vi "Execute.vi"(8 "error in (no error)":errorcluster, 10 "ObserverRegistry in":refnum<class "ObserverRegistry.lvclass">, 11 "ObserverRegistryCommand":refnum<class "Observer_RegisterForErrors.lvclass">) -> (0 "error out":errorcluster, 2 "ObserverRegistry out":refnum<class "ObserverRegistry.lvclass">, 3 "Message":refnum<class "MSG.lvclass">)   [LabVIEW 2011, in "Messenging.lvlib" / "Observer_RegisterForErrors.lvclass"]
uses:
  Observer_RegisterForErrors.lvclass
  ObserverRegistry.lvclass
  Interprocess Messenger/TextVarientMessage/MSG.lvclass
  Interprocess Messenger/SendMultiple/Create Observer.vi
  ParentCommand/ObserverRegistryCommand.lvclass
  Messenging.lvlib
  Interprocess Messenger/SendMultiple/ObserverSet.lvclass
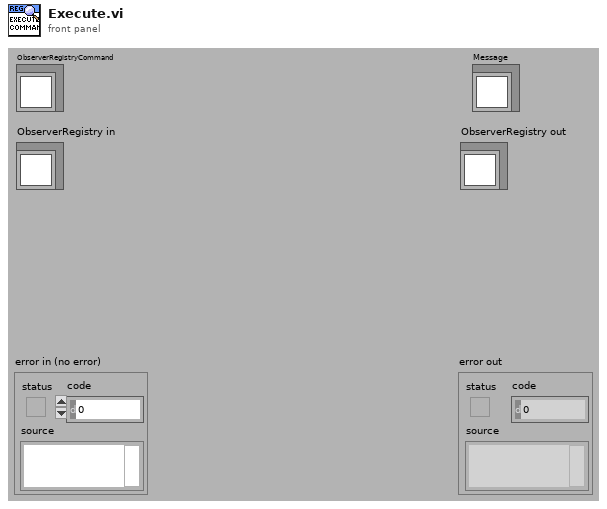
[diagram p1: front panel]
types:
  T1 = typedef "Messenging.lvlib/ObserverRegistry.lvclass/ObserverRegistryData.ctl" = cluster{"Observer of Errors":refnum<class "Observer.lvclass">, "Observer of All":refnum<class "Observer.lvclass">, "Event Registry":variant}
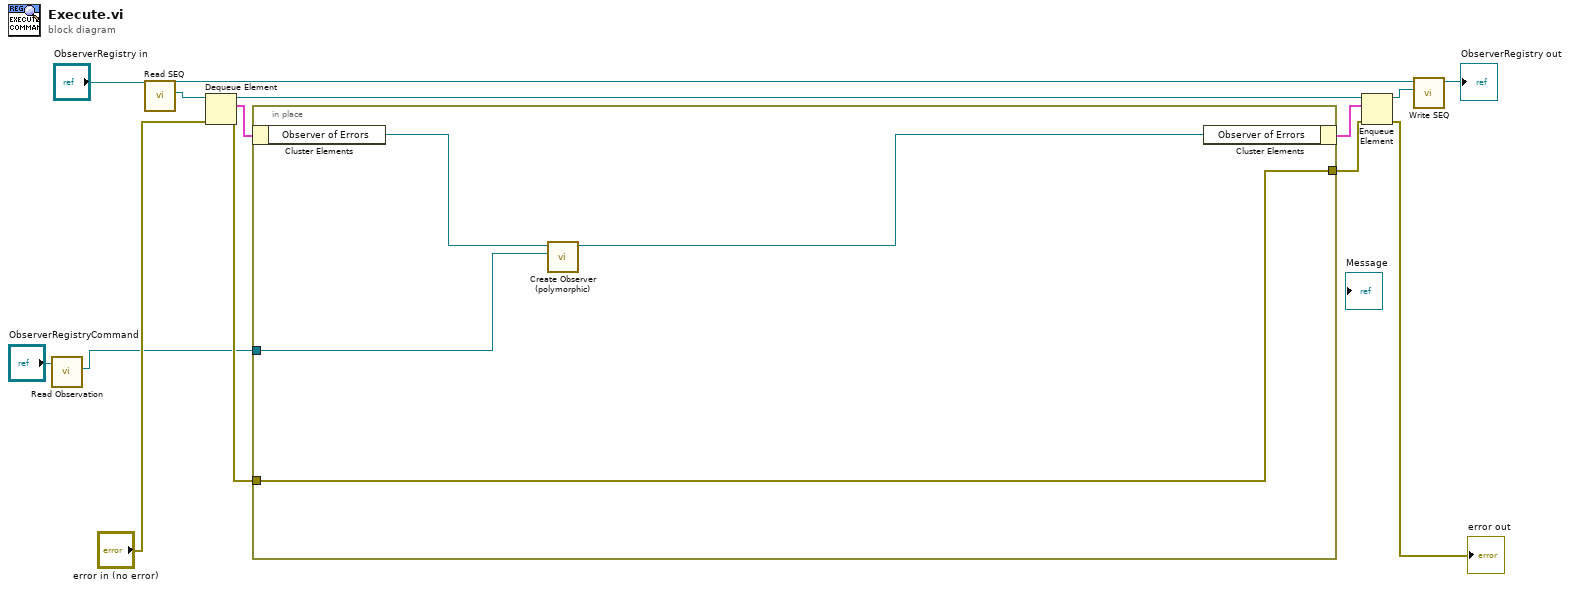
[diagram p0: block diagram]
diagram:
  n1 = call "Read Observation.vi"("ObserverRegistryCommand.lvclass in"="ObserverRegistryCommand") -> ("Observer"=w1:refnum<class "Send.lvclass">)  [unwired: 1 in, 9 out]
  n2 = call "Read SEQ.vi"("ObserverRegistry.lvclass in"="ObserverRegistry in") -> ("SEQ"=w7:refnum<queue>, "ObserverRegistry.lvclass out"=w5:refnum<class "ObserverRegistry.lvclass">)  [unwired: 1 in, 8 out]
  n3 = Dequeue Element(queue=w7, error in (no error)="error in (no error)") -> (queue out=w12:refnum<queue>, element=w14:T1, error out=w10:errorcluster)  [unwired: 2 out]
  n4 = in-place {
    in-place-border: w10 -> [w15]
    in-place-border: w1 -> [w17]
    in-place-border: [w15] -> w2
    n5 = in-place-cluster #1(w14) -> ("Observer of Errors"=w18:refnum<class "Observer.lvclass">)
    n6 = call-poly "Create Observer (polymorphic).vi"("Additional Input"=w17, "Input"=w18) -> ("Observer"=w16:refnum<class "Observer.lvclass">)  [unwired: 7 out]
    n7 = in-place-cluster #1("Observer of Errors"=w16) -> (w13:T1)
  }
  n8 = Enqueue Element(queue=w12, element=w13, error in (no error)=w2) -> (queue out=w4:refnum<queue>, error out=→"error out":errorcluster)  [unwired: 2 out]
  n9 = call "Write SEQ.vi"("SEQ"=w4, "ObserverRegistry.lvclass in"=w5) -> ("ObserverRegistry.lvclass out"=→"ObserverRegistry out":refnum<class "ObserverRegistry.lvclass">)  [unwired: 1 in, 8 out]
